vi "Show Windows(Security).vi"(10 "Mode String":string="Supervisor ", 11 "Message Reflesh Time":i16=3000) -> ()   [LabVIEW 2015]
panel:
  # "您已進入"
  # "家Α!"
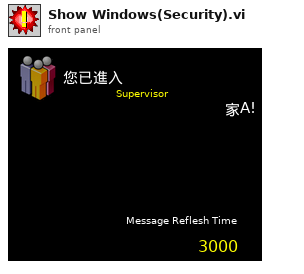
[diagram p1: front panel]
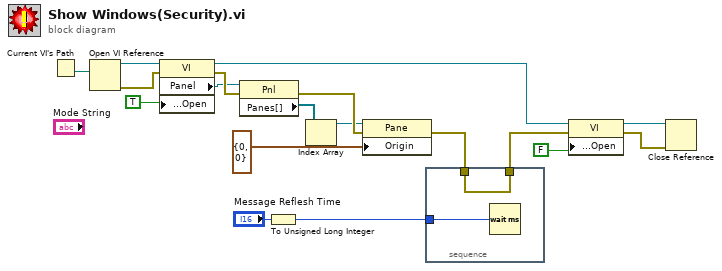
[diagram p0: block diagram]
diagram:
  n1 = Current VI's Path() -> (path=w16:path)
  n2 = Open VI Reference(vi path=w16) -> (vi reference=w10:refnum<vi>, error out=w11:errorcluster)  [unwired: 5 in]
  n3 = property class="VI"(reference=w10, error in=w11, "Front Panel.Open"=TRUE ("Front Panel Window:Open")) -> (reference out=w7:refnum<vi>, error out=w17:errorcluster, "Panel"=w15:refnum<vi>)
  n4 = property class="Pnl"(reference=w15, error in=w17) -> (error out=w18:errorcluster, "Panes[]"=w12:refnum<vi>[])  [unwired: 1 out]
  n5 = To Unsigned Long Integer(number="Message Reflesh Time") -> (unsigned 32bit integer=w1:u32)
  n6 = Index Array(array=w12) -> (element=w13:refnum<vi>)  [unwired: 1 in]
  n7 = property class="Pane"(reference=w13, error in=w18, "Origin"=cluster{"Horizontal":i16, "Vertical":i16} {"Horizontal"=0, "Vertical"=0}) -> (error out=w8:errorcluster)  [unwired: 1 out]
  n8 = stacked-sequence {
    tunnel: [w20] -> w4
    tunnel: w8 -> [w20]
    tunnel: w1 -> [w19]
    frame #0 {
      n9 = Wait (ms)(milliseconds to wait=w19) -> ()  [unwired: 1 out]
    }
  }
  n10 = property class="VI"(reference=w7, error in=w4, "Front Panel.Open"=FALSE ("Front Panel Window:Open")) -> (reference out=w6:refnum<vi>, error out=w3:errorcluster)
  n11 = Close Reference(reference=w6, error in (no error)=w3) -> ()  [unwired: 1 out]
